vi "Alert.vi"(5 "milliseconds to wait":u32=3000) -> ()   [LabVIEW 2020]
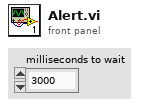
[diagram p1: front panel]
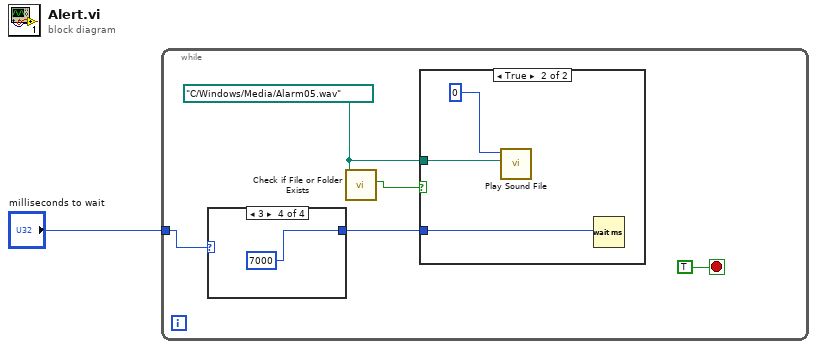
[diagram p0: block diagram]
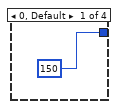
[diagram p2: hidden frame]
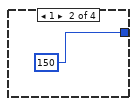
[diagram p3: hidden frame]
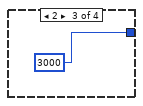
[diagram p4: hidden frame]
diagram:
  n1 = while {
    tunnel: "milliseconds to wait" -> [w3]
    stop <- TRUE stop-if-true
    w5 = path "C:/Windows/Media/Alarm05.wav"
    n2 = case shown="3" w3 {
      tunnel: [u32 150 ("milliseconds to wait") u32 150 ("milliseconds to wait") u32 3000 ("milliseconds to wait") u32 7000 ("milliseconds to wait")] -> w2
      frame 0, Default {
      }
      frame 1 {
      }
      frame 2 {
      }
      frame 3 {
      }
    }
    n3 = call <vilib>:"Check if File or Folder Exists.vi"("path"=w5) -> ("file or folder exists?"=w4:bool)  [unwired: 8 in, 2 out]
    n4 = case shown="True" w4 {
      tunnel: w5 -> [_ w12]
      tunnel: w2 -> [_ w11]
      frame False {
      }
      frame True {
        n5 = call <vilib>:"Play Sound File.vi"("path"=w12, "device ID"=u32 0) -> ()  [unwired: 8 in, 2 out]
        n6 = Wait (ms)(milliseconds to wait=w11) -> ()  [unwired: 1 out]
      }
    }
  }
